vi "MQTT_UnsubAck_Send.vi"(8 "error in (no error)":errorcluster, 10 "Message ID":u16=10 format="%x") -> (0 "error out":errorcluster, 2 "UnSuback Message":u8[](array[numeric]) format="%x")   [LabVIEW 2019, in "MQTT_Functions.lvlib"]
uses:
  MQTT_Functions.lvlib
  Controls/MessageType.ctl
  Controls/Retain_Flag.ctl
  Controls/DUP_Flag.ctl
  Controls/QoS.ctl
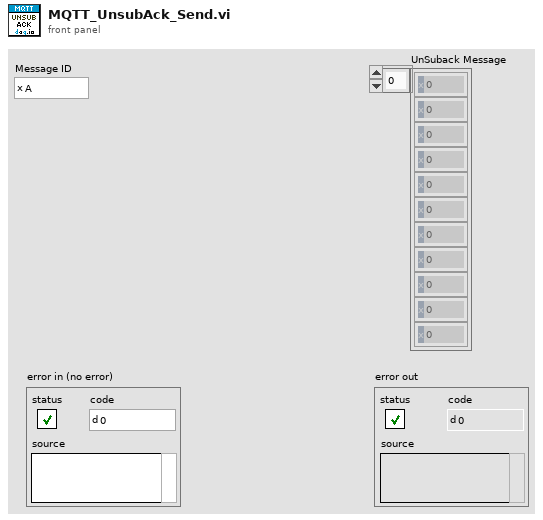
[diagram p1: front panel]
types:
  T1 = typedef "MQTT_Functions.lvlib/QoS.ctl" = enum8{"At most once", "At least once", "Exactly once", "Reserved"}
  T2 = typedef "MQTT_Functions.lvlib/DUP_Flag.ctl" = bool
  T3 = typedef "MQTT_Functions.lvlib/Retain_Flag.ctl" = bool
  T4 = typedef "MQTT_Functions.lvlib/MessageType.ctl" = enum32{"Reserved", "CONNECT", "CONNACK", "PUBLISH", "PUBACK", "PUBREC", "PUBREL", "PUBCOMP", "SUBSCRIBE", "SUBACK", "UNSUBSCRIBE", "UNSUBACK", "PINGREQ", "PINGRESP", "DISCONNECT", "Reserved2"}
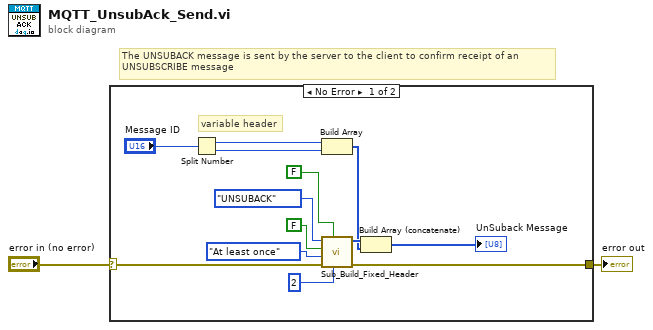
[diagram p0: block diagram]
diagram:
  # "The UNSUBACK message is sent by the server to the client to confirm receipt of an\nUNSUBSCRIBE message"
  n1 = case shown="No Error" "error in (no error)" {
    selector: "error in (no error)" -> [w4 w16]
    tunnel: [w14 w16] -> w1
    frame No Error {
      # "variable header"
      n2 = Split Number(x="Message ID") -> (hi(x)=w11:u8, lo(x)=w10:u8)
      n3 = Build Array(w11, w10) -> (w3:u8[])
      n4 = call "Sub_Build_Fixed_Header.vi"("Remaining Length"=u32 2, "Retain"=T3 FALSE, "error in (no error)"=w4, "QoS"=QoS."At least once", "DUP"=T2 FALSE, "MessageType"=MessageType."UNSUBACK") -> ("error out"=w14:errorcluster, "Fixed Header"=w13:u8[])  [unwired: 4 in]
      n5 = Build Array (concatenate)(w13, w3) -> (→"UnSuback Message":u8[])
    }
    frame Error {
    }
  }
  "error out" <- w1
